vi "Test camera initialization.vi"() -> ()   [LabVIEW 2020]
uses:
  <vilib>/userdefined/High Color/IMAQdx.ctl
  <vilib>/vision/driver/NI_Vision_Acquisition_Software.lvlib
panel:
  out "Image":T1(plugin-control)
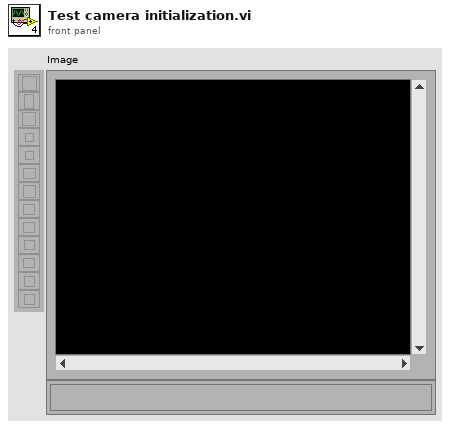
[diagram p1: front panel]
types:
  T1 = typedef "IMAQ Image.ctl" = refnum<image>
  T2 = typedef "IMAQdx.ctl" = refnum<k21>
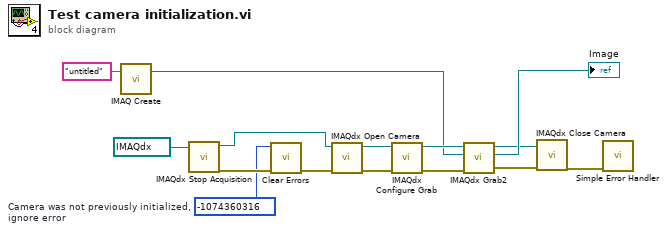
[diagram p0: block diagram]
diagram:
  w1 = -1074360316  # Camera was not previously initialized, ignore error
  n1 = call "IMAQ Create"("Image Name"="untitled") -> ("New Image"=w10:T1)  [unwired: 4 in, 1 out]
  n2 = call <vilib>:"IMAQdx Stop Acquisition.vi"("Session In"=T2 "cam0") -> ("error out"=w4:errorcluster, "Session Out"=w2:T2)  [unwired: 9 in]
  n3 = call <vilib>:"Clear Errors.vi"("error in (no error)"=w4, "specific error code to clear (0: all)"=w1) -> ("error out"=w3:errorcluster)  [unwired: 4 in, 1 out]
  n4 = call <vilib>:"IMAQdx Open Camera.vi"("error in"=w3, "Session In"=w2) -> ("error out"=w6:errorcluster, "Session Out"=w7:T2)  [unwired: 8 in]
  n5 = call <vilib>:"IMAQdx Configure Grab.vi"("error in"=w6, "Session In"=w7) -> ("error out"=w15:errorcluster, "Session Out"=w14:T2)  [unwired: 8 in]
  n6 = call <vilib>:"IMAQdx Grab2.vi"("error in"=w15, "Image In"=w10, "Session In"=w14) -> ("error out"=w12:errorcluster, "Image Out"=→"Image":T1, "Session Out"=w11:T2)  [unwired: 5 in, 1 out]
  n7 = call <vilib>:"IMAQdx Close Camera.vi"("error in"=w12, "Session In"=w11) -> ("error out"=w8:errorcluster)  [unwired: 9 in]
  n8 = call <vilib>:"Simple Error Handler.vi"("error in (no error)"=w8) -> ()  [unwired: 4 in, 5 out]
